vi "Init.vi"(8 "error in":errorcluster, 11 "DAQmx Base Configure Strategy in":refnum<class "DAQmx Base Configure Strategy.lvclass">) -> (0 "error out":errorcluster, 3 "DAQmx Base Configure Strategy out":refnum<class "DAQmx Base Configure Strategy.lvclass">)   [LabVIEW 2024, in "DAQmx Base Configure Strategy.lvclass"]
uses:
  DAQmx Base Configure Strategy.lvclass
  DAQmx Base Configure Strategy.lvclass/DAQmx Base Configure Strategy.ctl
  Source/Interfaces/IConfiguration/IConfiguration.lvclass
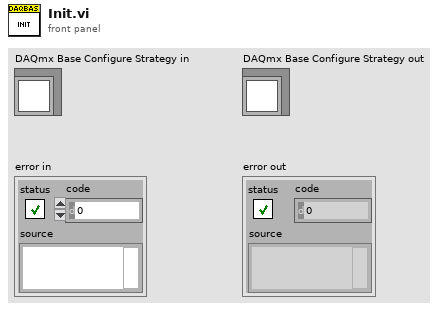
[diagram p1: front panel]
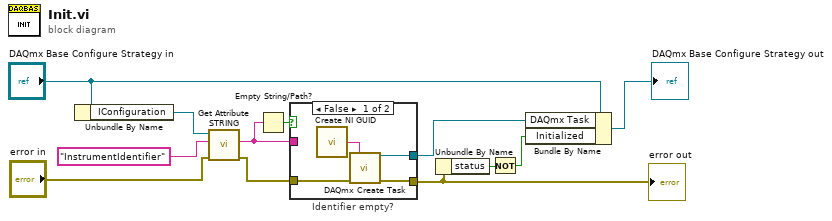
[diagram p0: block diagram]
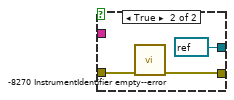
[diagram p2: hidden frame]
diagram:
  n1 = Unbundle By Name("DAQmx Base Configure Strategy in") -> ("IConfiguration"=w10:refnum<class "IConfiguration.lvclass">)
  n2 = call-dynamic "Get Attribute STRING.vi"("error in"="error in", "Attribute"="InstrumentIdentifier", "IConfiguration in"=w10) -> ("error out"=w5:errorcluster, "Value"=w4:string)  [unwired: 6 in, 1 out]
  n3 = Empty String/Path?(string/path=w4) -> (empty?=w12:bool)
  n4 = case "Identifier empty?" shown="False" w12 {
    tunnel: w5 -> [w13 w18]
    tunnel: [w16 w17] -> w3
    tunnel: [w14 refnum<k21> refnum ("task out")] -> w11
    tunnel: w4 -> [_ _]
    frame False {
      n5 = call <vilib>:"Create NI GUID.vi"() -> ("NI GUID"=w15:string)
      n6 = call <vilib>:"DAQmx Create Task.vi"("new task name"=w15, "error in"=w13) -> ("task out"=w14:refnum<k21>, "error out"=w16:errorcluster)  [unwired: 12 in]
    }
    frame True {
      n7 = call "-8270 InstrumentIdentifier empty--error.vi"("error in"=w18) -> ("error out"=w17:errorcluster)  [unwired: 10 in]
    }
  }
  "error out" <- w3
  n8 = Unbundle By Name(w3) -> ("status"=w2:bool)
  n9 = Not(x=w2) -> (.not. x?=w1:bool)
  n10 = Bundle By Name(cluster="DAQmx Base Configure Strategy in", "DAQmx Task"=w11, "Initialized"=w1) -> (→"DAQmx Base Configure Strategy out":refnum<class "DAQmx Base Configure Strategy.lvclass">)
